vi "Insert Case Structure.vi"(0 "Test Executive in":refnum<class "Test Executive.lvclass">, 1 "Name":string, 2 "Unique ID":string, 3 "Insertion Index":i32=-1, 4 "Assertions":refnum<class "Assert.lvclass">[](array[class]), 5 "error in (no error)":errorcluster, 6 "Parent ID":string, 7 "X Variables":string[](array[string]), 9 "Y Variables":string[](array[string]), 11 "Conditional Branches":string[](array[string]), 13 "\"Else\" Conditional Branch":string) -> (12 "Unique ID out":string, 14 "Test Executive out":refnum<class "Test Executive.lvclass">, 17 "Replaced?":bool, 19 "error out":errorcluster)   [LabVIEW 2020, in "Test Executive.lvlib" / "Test Executive.lvclass"]
uses:
  <vilib>/gpm_packages/@cs/test-executive/Source/Test Executive/TestExecutive/Test Executive.lvclass
  <vilib>/gpm_packages/@cs/run-time-assertions/Source/Assert/Assert.lvclass
  <vilib>/gpm_packages/@cs/test-executive/Source/Test Executive/Case Structure/Case Structure.lvclass
  <vilib>/gpm_packages/@cs/test-executive/Source/Test Executive/TestExecutive/Test Executive.lvclass/Test Executive.ctl
  06cb589e-ef21-4d9c-bc6f-c44a03bd748f.vi
  41ee88d5-44eb-43c1-be10-d5447cb375ae.vi
  8f35472b-3519-4b8d-80db-249a6bffe38d.vi
  50cad2ab-e04f-4e73-935b-b825fae1b99f.vi
  7b87c44f-d849-49bd-9ca1-cbb741886ff0.vi
  bff56f29-40a7-479f-8d84-a2f932ece95c.vi
  37040775-d56e-4ea4-86e9-01ed9cceefda.vi
  <vilib>/gpm_packages/@cs/linked-list/Source/Linked List/ILinkedList/ILinked List.lvclass
  <vilib>/gpm_packages/@cs/linked-list/Source/Linked List/Linked List Ref/Linked List Ref.lvclass
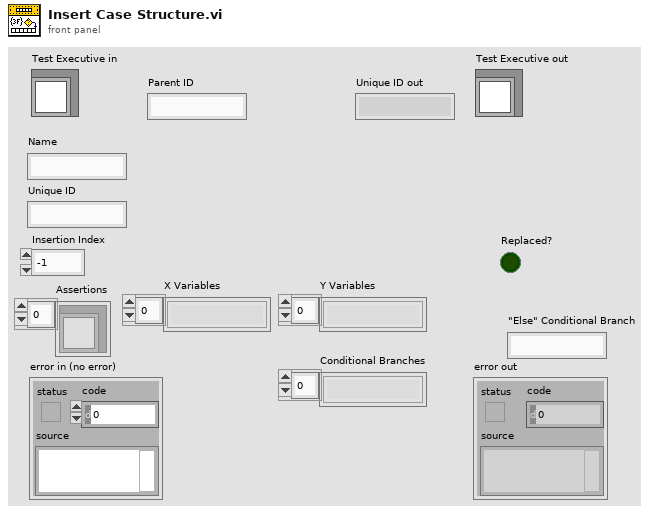
[diagram p1: front panel]
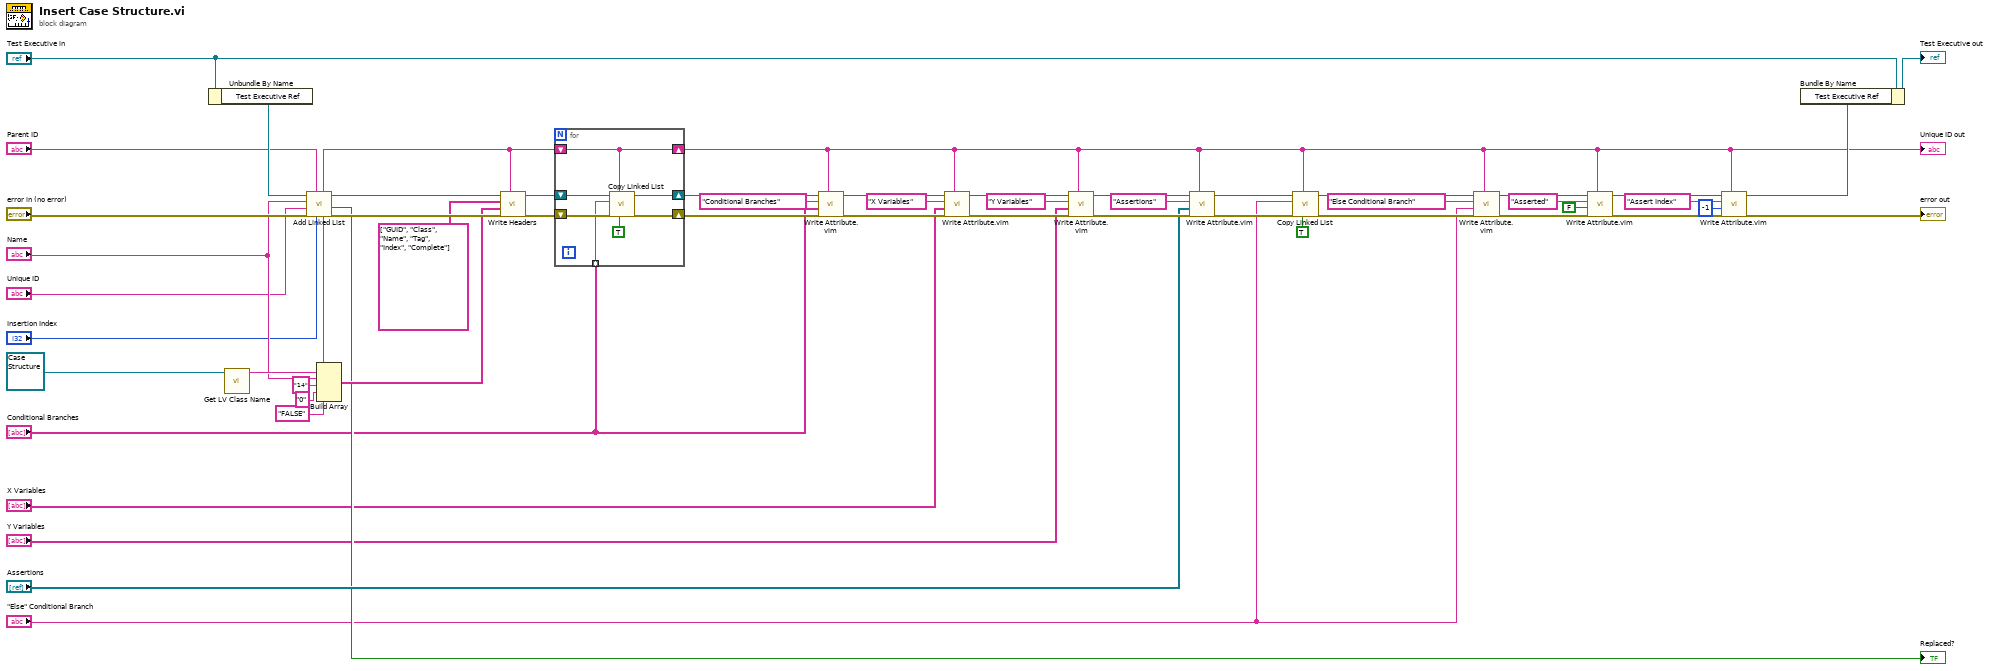
[diagram p0: block diagram]
diagram:
  n1 = Unbundle By Name("Test Executive in") -> ("Test Executive Ref"=w55:refnum<data-value>)
  n2 = call <vilib>:"Get LV Class Name.vi"("object"=refnum<class "Case Structure.lvclass"> refnum ("Test Executive.lvlib:Case Structure.lvclass")) -> ("class name"=w51:string)  [unwired: 9 in, 1 out]
  n3 = call <vilib>:"Add Linked List.vi"("Insertion Index"="Insertion Index", "Parent ID"="Parent ID", "error in (no error)"="error in (no error)", "Linked List ID"="Unique ID", "Name"="Name", "Linked List Ref"=w55) -> ("error out"=w53:errorcluster, "Replaced?"=→"Replaced?":bool, "Linked List Ref out"=w54:refnum<data-value>, "Linked List ID out"=w19:string)  [unwired: 2 in]
  n4 = Build Array(w19, w51, "Name", "14" ("element"), "0" ("element"), "FALSE" ("element")) -> (w49:string[])
  n5 = call <vilib>:"Write Headers.vi"("Linked List ID"=w19, "error in (no error)"=w53, "Header Values"=w49, "Header Names"=string[] ["GUID", "Class", "Name", "Tag", "Index", "Complete"], "Linked List Ref"=w54) -> ("error out"=w47:errorcluster, "Linked List Ref out"=w48:refnum<data-value>)  [unwired: 5 in]
  n6 = for {
    tunnel: "Conditional Branches" -> [w57] mode=indexing
    shift-right: [w59] -> w17
    shift-left: w48 -> [w62]
    shift-right: [w58] -> w16
    shift-left: w47 -> [w61]
    shift-right: [w56] -> w2
    shift-left: w19 -> [w56]
    n7 = call <vilib>:"Copy Linked List.vi"("Move?"=TRUE, "New Parent Linked List ID"=w56, "error in (no error)"=w61, "Linked List ID"=w57, "Linked List Ref"=w62) -> ("error out"=w58:errorcluster, "Linked List Ref out"=w59:refnum<data-value>)  [unwired: 3 in, 2 out]
  }
  "Unique ID out" <- w2
  n8 = call "Write Attribute.vim"("Linked List ID"=w2, "error in (no error)"=w16, "Attribute"="Conditional Branches", "Attribute Name"="Conditional Branches", "Linked List Ref"=w17) -> ("error out"=w14:errorcluster, "Linked List Ref out"=w15:refnum<data-value>)  [unwired: 3 in, 2 out]
  n9 = call "Write Attribute.vim"("Linked List ID"=w2, "error in (no error)"=w14, "Attribute"="X Variables", "Attribute Name"="X Variables", "Linked List Ref"=w15) -> ("error out"=w43:errorcluster, "Linked List Ref out"=w44:refnum<data-value>)  [unwired: 3 in, 2 out]
  n10 = call "Write Attribute.vim"("Linked List ID"=w2, "error in (no error)"=w43, "Attribute"="Y Variables", "Attribute Name"="Y Variables", "Linked List Ref"=w44) -> ("error out"=w40:errorcluster, "Linked List Ref out"=w41:refnum<data-value>)  [unwired: 3 in, 2 out]
  n11 = call "Write Attribute.vim"("Linked List ID"=w2, "error in (no error)"=w40, "Attribute"="Assertions", "Attribute Name"="Assertions", "Linked List Ref"=w41) -> ("error out"=w4:errorcluster, "Linked List Ref out"=w6:refnum<data-value>)  [unwired: 3 in, 2 out]
  n12 = call <vilib>:"Copy Linked List.vi"("Move?"=TRUE, "New Parent Linked List ID"=w2, "error in (no error)"=w4, "Linked List ID"="\"Else\" Conditional Branch", "Linked List Ref"=w6) -> ("error out"=w3:errorcluster, "Linked List Ref out"=w5:refnum<data-value>)  [unwired: 3 in, 2 out]
  n13 = call "Write Attribute.vim"("Linked List ID"=w2, "error in (no error)"=w3, "Attribute"="\"Else\" Conditional Branch", "Attribute Name"="Else Conditional Branch", "Linked List Ref"=w5) -> ("error out"=w9:errorcluster, "Linked List Ref out"=w10:refnum<data-value>)  [unwired: 3 in, 2 out]
  n14 = call "Write Attribute.vim"("Linked List ID"=w2, "error in (no error)"=w9, "Attribute"=FALSE, "Attribute Name"="Asserted", "Linked List Ref"=w10) -> ("error out"=w34:errorcluster, "Linked List Ref out"=w35:refnum<data-value>)  [unwired: 3 in, 2 out]
  n15 = call "Write Attribute.vim"("Linked List ID"=w2, "error in (no error)"=w34, "Attribute"=-1, "Attribute Name"="Assert Index", "Linked List Ref"=w35) -> ("error out"=→"error out":errorcluster, "Linked List Ref out"=w32:refnum<data-value>)  [unwired: 3 in, 2 out]
  n16 = Bundle By Name(cluster="Test Executive in", "Test Executive Ref"=w32) -> (→"Test Executive out":refnum<class "Test Executive.lvclass">)
